vi "Expr_Send LIN Uncond Frame.vi"(0 "Toolkit Type":enum16{"Inalfa LIN", "ADCS LIN", "TS LIN"}(ring), 1 "data string":string, 2 "byte log":string, 5 "Inalfa LIN":T2={"Master Frame(3C)"="MasterReq\nSPA3414_ConfigurationsCMAGeely_CEMCALYPSOSDB34XX0Cfg_LIN3_190709_", "Slave Frame(3D)"="SlaveResp\nSPA3414_ConfigurationsCMAGeely_CEMCALYPSOSDB34XX0Cfg_LIN3_190709_", "Request Schedule"="CEMLIN3DiagRequestSchedule\nSPA3414_ConfigurationsCMAGeely_CEMCALYPSOSDB34XX0Cfg_LIN3_190709_", "Response Schedule"="CEMLIN3DiagResponseSchedule\nSPA3414_ConfigurationsCMAGeely_CEMCALYPSOSDB34XX0Cfg_LIN3_190709_", "Frame Write SCU"="", "Frame Read SCU"="", "LIN Name"=""}, 7 "TS LIN":T4, 9 "ADCS LIN":T1={"Port"="LIN1", "HW select"=0, "XNET Cluster"="NIXNET_exampleLDF", "ByteCmd Path"=path "C:/Labview Code/System/ByteCmdConfig.txt"} {"HW select" items=["NI-XNET", "NI-CAN"]}, 11 "error in":errorcluster caption="错误常量", 12 "Current Motion":T3=enum."Express Sunshade Close") -> (6 "byte log":string, 15 "error out":errorcluster)   [LabVIEW 2018]
uses:
  C:/Program Files (x86)/National Instruments/LabVIEW 2018/vi.lib/CMC.AME/Inalfa TS LIN/TOSUN/TSMaster/bin/Interop.TSMasterAPI.dll
  Program Files (x86)/National Instruments/LabVIEW 2018/vi.lib/CMC.AME/Inalfa TS LIN/TOSUN/TSMaster/bin/Interop.TSMasterAPI.dll
  02.Type Def's/All Motions.ctl
  03.Inalfa LIN/LIN Device.ctl
  <vilib>/CMC.AME/Inalfa ADCS/Ctl'Def/ADCS_LIN info.ctl
  05.UserVI's/type defs/17x Audit Motion Data Seq Control.ctl
  05.UserVI's/type defs/17x AP Data Type.ctl
  <vilib>/xnet/xnet.llb/XNET Frame LIN.ctl
  <vilib>/xnet/xnet.llb/XNET Frame Type LIN.ctl
  <vilib>/xnet/xnet.llb/XNET Create Session (Frame Output Stream).vi
  <vilib>/xnet/xnet.llb/XNET Write (Frame LIN).vi
  <resource>/objmgr/xnet.rc
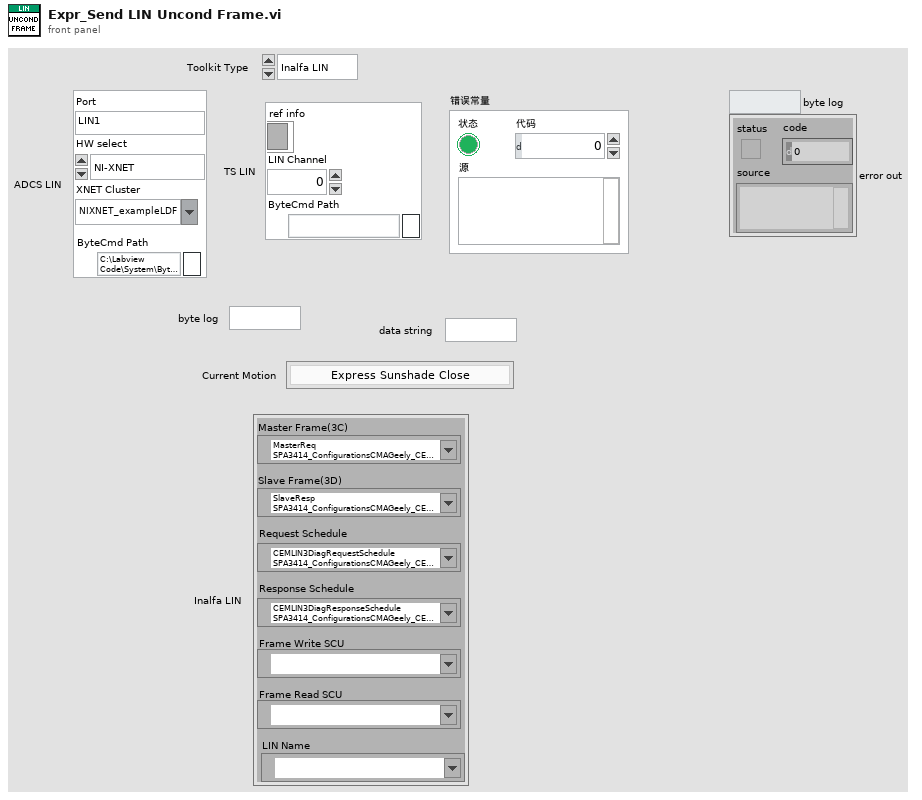
[diagram p1: front panel]
types:
  T1 = typedef "ADCS_LIN info.ctl" = cluster{"Port":string, "HW select":u16, "XNET Cluster":string, "ByteCmd Path":path}
  T2 = typedef "LIN Device.ctl" = cluster{"Master Frame(3C)":refnum<k21>, "Slave Frame(3D)":refnum<k21>, "Request Schedule":refnum<k21>, "Response Schedule":refnum<k21>, "Frame Write SCU":refnum<k21>, "Frame Read SCU":refnum<k21>, "LIN Name":refnum<k21>}
  T3 = typedef "All Motions.ctl" = enum16{"Glass Teach", "Glass Slide Open", "Glass Slide Close", "Glass Vent Open", "Glass Vent Close", "Sunshade Teach", "Sunshade Open", "Sunshade Close", "Idle", "Sunshade Open 2", "Sunshade Close 2", "Glass Slide Open Sunshade Open", "Glass Slide Open Sunshade Close", "Glass Slide Close Sunshade Open", "Glass Slide Close Sunshade Close", "Glass Vent Open Sunshade Open", "Glass Vent Open Sunshade Close", "Glass Vent Close Sunshade Open", "Glass Vent Close Sunshade Close", "Express Glass Slide Open", "Express Glass Slide Close", "Express Glass Vent Open", "Express Glass Vent Close", "Express Sunshade Open", "Express Sunshade Close", "Express Sunshade Open 2", "Express Sunshade Close 2", "Express Glass Slide Open Sunshade Open", "Express Glass Slide Open Sunshade Close", "Express Glass Slide Close Sunshade Open", "Express Glass Slide Close Sunshade Close", "Express Glass Vent Open Sunshade Open", "Express Glass Vent Open Sunshade Close", "Express Glass Vent Close Sunshade Open", "Express Glass Vent Close Sunshade Close", "Goto Position Glass", "Goto Position Sunshade", "Sunshade Teach 2"}
  T4 = cluster{"ref info":refnum<k24>, "LIN Channel":i32, "ByteCmd Path":path}
  T5 = typedef "17x Audit Motion Data Seq Control.ctl" = cluster{"Power Supply Voltage":dbl, "Min Avg Current":dbl, "Max Avg Current":dbl, "Min Run Time":dbl, "Max Run Time":dbl, "Min Speed":dbl, "Max Speed":dbl, "AP Data % of Threshold":dbl, "Travel Distance":dbl, "AP Data Type":T6, "Check Current":bool, "Check Run Time":bool, "Check Speed":bool, "Express Motion?":bool, "Check Sound Test":bool, "Check Position?":bool, "Collect AP Data":bool, "Inital Position":u16, "End Position":u16, "Goto Posiition":u16, "Max max Current":dbl, "Min max Current":dbl, "Check max Current":bool, "Check Sound":bool, "Min Sound (dB)":dbl, "Max Sound (dB)":dbl, "SW Mode":enum16{"Hard Switch", "Uncond Frame"}, "LIN Msg":cluster{"ID":u8, "Msg":u8[][], "LDF":refnum<k21>}}
  T6 = typedef "17x AP Data Type.ctl" = enum16{"91/61", "92/62", "93/63", "67", "68", "6F", "71", "91 Msg", "92 Msg", "93 Msg", "94 Msg", "HiRain 91", "HiRain 92 Speed", "HiRain 92 HS", "HiRain 92", "HiRain 93", "SnT"}
  T7 = typedef "XNET Frame LIN.ctl" = cluster{"timestamp":timestamp, "payload":u8[], "identifier":u32, "type":T8, "event ID":u8, "event slot?":bool, "echo?":bool}
  T8 = typedef "XNET Frame Type LIN.ctl" = u8
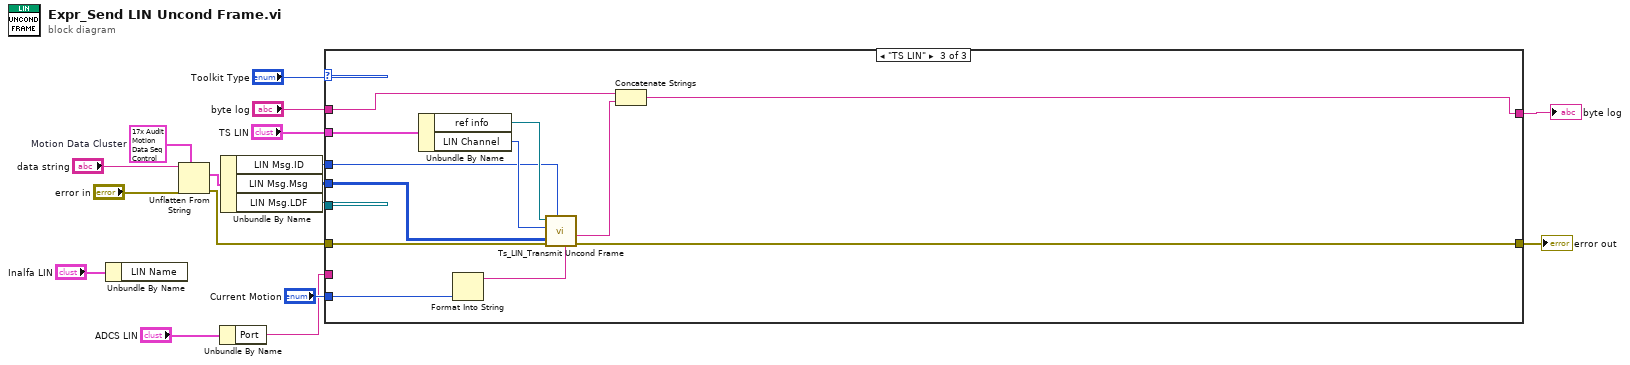
[diagram p0: block diagram]
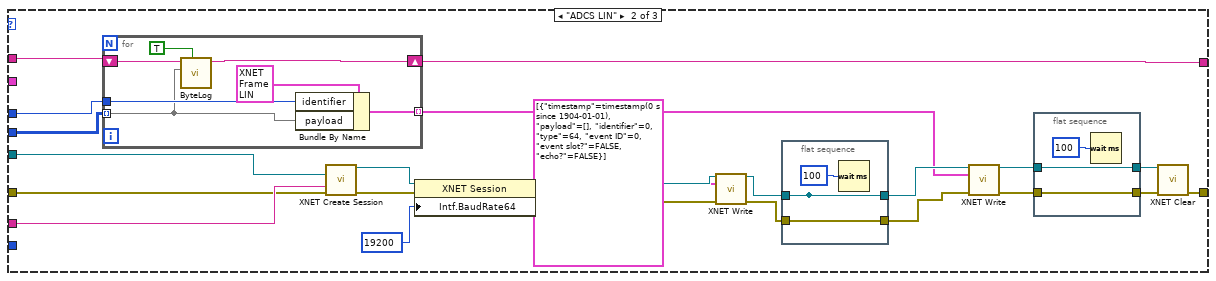
[diagram p3: hidden frame]
diagram:
  w14 = T5 {"Power Supply Voltage"=0.0, "Min Avg Current"=0.0, "Max Avg Current"=0.0, "Min Run Time"=0.0, "Max Run Time"=0.0, "Min Speed"=0.0, "Max Speed"=0.0, "AP Data % of Threshold"=0.0, "Travel Distance"=0.0, "AP Data Type"=enum."91/61", "Check Current"=FALSE, "Check Run Time"=FALSE, "Check Speed"=FALSE, "Express Motion?"=FALSE, "Check Sound Test"=FALSE, "Check Position?"=FALSE, "Collect AP Data"=FALSE, "Inital Position"=0, "End Position"=0, "Goto Posiition"=0, "Max max Current"=0.0, "Min max Current"=0.0, "Check max Current"=FALSE, "Check Sound"=FALSE, "Min Sound (dB)"=0.0, "Max Sound (dB)"=0.0, "SW Mode"=enum."Hard Switch", "LIN Msg"={"ID"=0, "Msg"=[], "LDF"="EX1H"}}  # Motion Data Cluster
  n1 = Unbundle By Name("Inalfa LIN") -> ()  [unwired: 1 out]
  n2 = Unflatten From String(type=w14, binary string="data string", error in (no error)="error in") -> (value=w13:T5, error out=w5:errorcluster)  [unwired: 2 in, 1 out]
  n3 = Unbundle By Name("ADCS LIN") -> ("Port"=w3:string)
  n4 = Unbundle By Name(w13) -> ("LIN Msg.ID"=w9:u8, "LIN Msg.Msg"=w10:u8[][], "LIN Msg.LDF"=w2:refnum<k21>)
  n5 = case shown="\"TS LIN\"" "Toolkit Type" {
    tunnel: "TS LIN" -> [_ _ w66]
    tunnel: w5 -> [w18 w30 w63]
    tunnel: "Current Motion" -> [_ _ w62]
    tunnel: [_ w20 w55] -> w11
    tunnel: w10 -> [_ w36 w61]
    tunnel: w9 -> [_ w37 w58]
    tunnel: w3 -> [_ w41 _]
    tunnel: [w18 w31 w60] -> w7
    tunnel: w2 -> [_ w22 _]
    tunnel: "byte log" -> [_ w19 w57]
    frame "Inalfa LIN", Default {
    }
    frame "ADCS LIN" {
      n6 = for {
        tunnel: w37 -> [w53]
        tunnel: w36 -> [w50] mode=indexing
        tunnel: [w52] -> w23 mode=indexing
        shift-right: [w48] -> w20
        shift-left: w19 -> [w49]
        n7 = call <vilib>:"ByteLog.vi"("Tx?"=TRUE, "byte"=w50, "byte log"=w49) -> ("byte log"=w48:string)  [unwired: 7 in, 1 out]
        n8 = Bundle By Name(cluster=T7 {"timestamp"=timestamp(0 s since 1904-01-01), "payload"=[], "identifier"=0, "type"=64, "event ID"=0, "event slot?"=FALSE, "echo?"=FALSE} ("LIN frame"), "identifier"=w53, "payload"=w50) -> (w52:T7)
      }
      n9 = call-poly <vilib>:"XNET Create Session.vi"("cluster (:memory:)"=w22, "interface"=w41, "error in (no error)"=w30) -> ("session out"=w40:refnum<k21>, "error out"=w38:errorcluster)  [unwired: 11 in]
      n10 = property class="XNET Session"(reference=w40, error in=w38, "Intf.BaudRate64"=u64 19200 ("Interface:64bit Baud Rate")) -> (reference out=w29:refnum<k21>, error out=w28:errorcluster)
      n11 = call-poly <vilib>:"XNET Write.vi"("session in"=w29, "data"=T7[] [{"timestamp"=timestamp(0 s since 1904-01-01), "payload"=[], "identifier"=0, "type"=64, "event ID"=0, "event slot?"=FALSE, "echo?"=FALSE}], "error in (no error)"=w28) -> ("session out"=w27:refnum<k21>, "error out"=w26:errorcluster)  [unwired: 11 in]
      n12 = flat-sequence {
        tunnel: w26 -> [w43]
        tunnel: [w43] -> w24
        tunnel: w27 -> [w42]
        tunnel: [w42] -> _
        tunnel: [w42] -> w25
        frame #0 {
          n13 = Wait (ms)(milliseconds to wait=u32 100 ("等待时间（毫秒）")) -> ()  [unwired: 1 out]
        }
      }
      n14 = call-poly <vilib>:"XNET Write.vi"("session in"=w25, "data"=w23, "error in (no error)"=w24) -> ("session out"=w33:refnum<k21>, "error out"=w35:errorcluster)  [unwired: 11 in]
      n15 = flat-sequence {
        tunnel: w35 -> [w46]
        tunnel: [w46] -> w34
        tunnel: w33 -> [w45]
        tunnel: [w45] -> w32
        frame #0 {
          n16 = Wait (ms)(milliseconds to wait=u32 100 ("等待时间（毫秒）")) -> ()  [unwired: 1 out]
        }
      }
      n17 = call <vilib>:"XNET Clear.vi"("session in"=w32, "error in (no error)"=w34) -> ("error out"=w31:errorcluster)  [unwired: 13 in]
    }
    frame "TS LIN" {
      n18 = Unbundle By Name(w66) -> ("ref info"=w65:refnum<k24>, "LIN Channel"=w64:i32)
      n19 = Format Into String(w62) -> (resulting string=w59:string)  [unwired: 3 in, 1 out]
      n20 = call <vilib>:"Ts_LIN_Transmit Uncond Frame.vi"("loop event"=w59, "Req Data"=w61, "FIdentifier"=w58, "错误输入（无错误）"=w63, "LIN Channel"=w64, "TsRef in"=w65) -> ("错误输出"=w60:errorcluster, "byte log"=w56:string)  [unwired: 3 in, 1 out]
      n21 = Concatenate Strings(w57, w56) -> (w55:string)
    }
  }
  "byte log" <- w11
  "error out" <- w7
